vi "OpenDataClassReference.vi"(8 "error in (no error)":errorcluster) -> (0 "error out":errorcluster, 3 "DataClassNotifier out":refnum<notifier>)   [LabVIEW 2013, in "Data.lvclass"]
uses:
  Data.lvclass
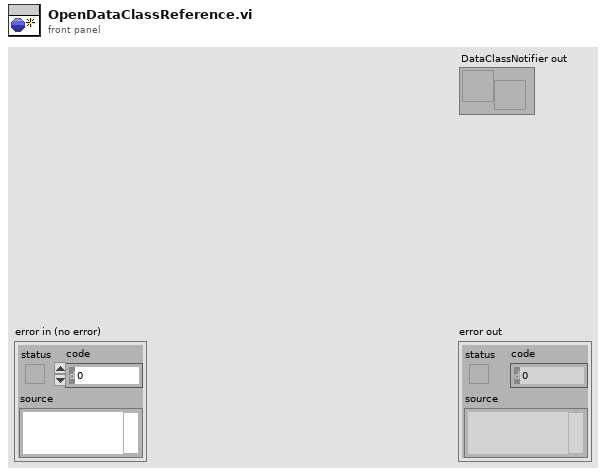
[diagram p1: front panel]
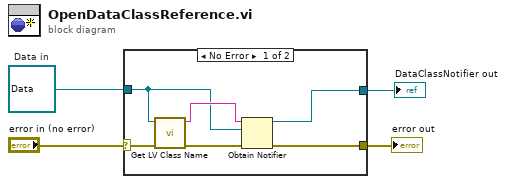
[diagram p0: block diagram]
diagram:
  w2 = refnum<class "Data.lvclass"> refnum  # Data in
  n1 = case shown="No Error" "error in (no error)" {
    selector: "error in (no error)" -> [w10 w11]
    tunnel: [w9 w11] -> w3
    tunnel: w2 -> [w6 _]
    tunnel: [w7 _] -> w1
    frame No Error {
      n2 = call <vilib>:"Get LV Class Name.vi"("error in (no error)"=w10, "object"=w6) -> ("error out"=w5:errorcluster, "class name"=w8:string)  [unwired: 8 in]
      n3 = Obtain Notifier(name (unnamed)=w8, notification data type=w6, error in (no error)=w5) -> (notifier out=w7:refnum<notifier>, error out=w9:errorcluster)  [unwired: 1 in, 1 out]
    }
    frame Error {
    }
  }
  "error out" <- w3
  "DataClassNotifier out" <- w1
